vi "RobotMain.vi"() -> ()   [LabVIEW 2014]
uses:
  Command.ctl
  DataHighway.ctl
  <vilib>/userdefined/High Color/IMAQdx.ctl
  <vilib>/myRIO/Common/Instrument Driver Framework/myRIO v1.0/UART/vis/myRIO v1.0 Close UART.vi
  <vilib>/myRIO/Common/Instrument Driver Framework/Utilities/vis/FPGA Ref Manager.vi
  <vilib>/myRIO/Common/Instrument Driver Framework/myRIO v1.0/myRIO v1.0 Reset FPGA.vi
  <vilib>/myRIO/Common/Instrument Driver Framework/myRIO v1.0/IRQ/vis/myRIO v1.0 IRQ Info FGV.vi
  <vilib>/myRIO/Common/Instrument Driver Framework/myRIO v1.0/IRQ/vis/myRIO v1.0 Timer IRQ Info FGV.vi
  <vilib>/myRIO/Common/Instrument Driver Framework/myRIO v1.0/IRQ/vis/myRIO v1.0 ISR Agent.vi
  <vilib>/ErrorRing/Error Ring.xnode
  <vilib>/myRIO/Instrument Drivers/Utilities/Utilities.lvlib
  <vilib>/vision/driver/NI_Vision_Acquisition_Software.lvlib
panel:
  out "Camera open ok?":errorcluster
  out "Robot Run ok":bool
  out "Color Image":T1(plugin-control)
  out "BW Image":T1(plugin-control)
  out "Nb Circles":i32
  out "Camera Data":T2(array[cluster])
  out "GPS":cluster{"X pos":i32, "Y pos":i32, "Heading":dbl}
  in  "Tug Letter":string="T"
  out "GPS OK?":bool
  out "DataHWay":T3
  out "ComHWayFromOCU":T4 {"Speed" scale=-2.0..10.0; "Rudder" scale=-10.0..10.0}
  in  "stop robot control":bool
  out "Final myRIO error":errorcluster
  # "set\nletter"
  # "Robot will run headless\nwithout a control panel\nso keep this control panel\nas simple as possible while\nstill allowing debugging."
  # "Data Highway carries all robot data"
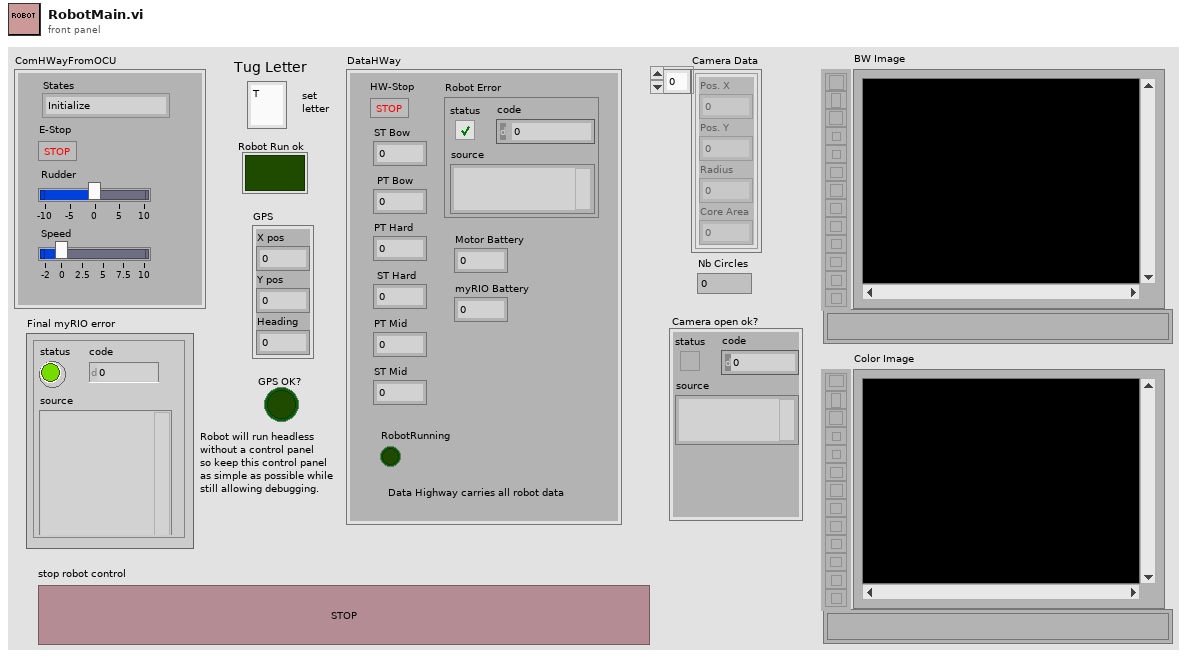
[diagram p1: front panel]
types:
  T1 = typedef "IMAQ Image.ctl" = refnum<image>
  T2 = cluster{"Pos. X":i32, "Pos. Y":i32, "Radius":i32, "Core Area":i32}[]
  T3 = typedef "DataHighway.ctl" = cluster{"HW-Stop":bool, "ST Bow":dbl, " PT Bow":dbl, "PT Hard":dbl, "RobotRunning":bool, "Robot Error":errorcluster, " ST Hard":dbl, "PT Mid":dbl, "ST Mid":dbl, "Motor Battery":dbl, "myRIO Battery":dbl}
  T4 = typedef "Command.ctl" = cluster{"States":enum16{"Initialize", "Wait for Event", "Debug Robot", "Run Robot", "Exit", "Plan"}, "E-Stop":bool, "Rudder":dbl, "Speed":dbl}
  T5 = typedef "IMAQdx.ctl" = refnum<k21>
  T6 = typedef "Image Type" = u32
  T7 = enum16{"Initialize", "Wait for Event", "Debug Robot", "Run Robot", "Exit"}
  T8 = enum16{"Initialize", "Wait for Event", "Debug Robot", "Run Robot", "Exit", "Plan"}
  T9 = cluster{"StarBow":dbl, "Portbow":dbl, "PortHard":dbl, "Starhard":dbl, "PortMid":dbl, "StarMid":dbl}
  T10 = cluster{"regular expression":string, i32, i32, i32}
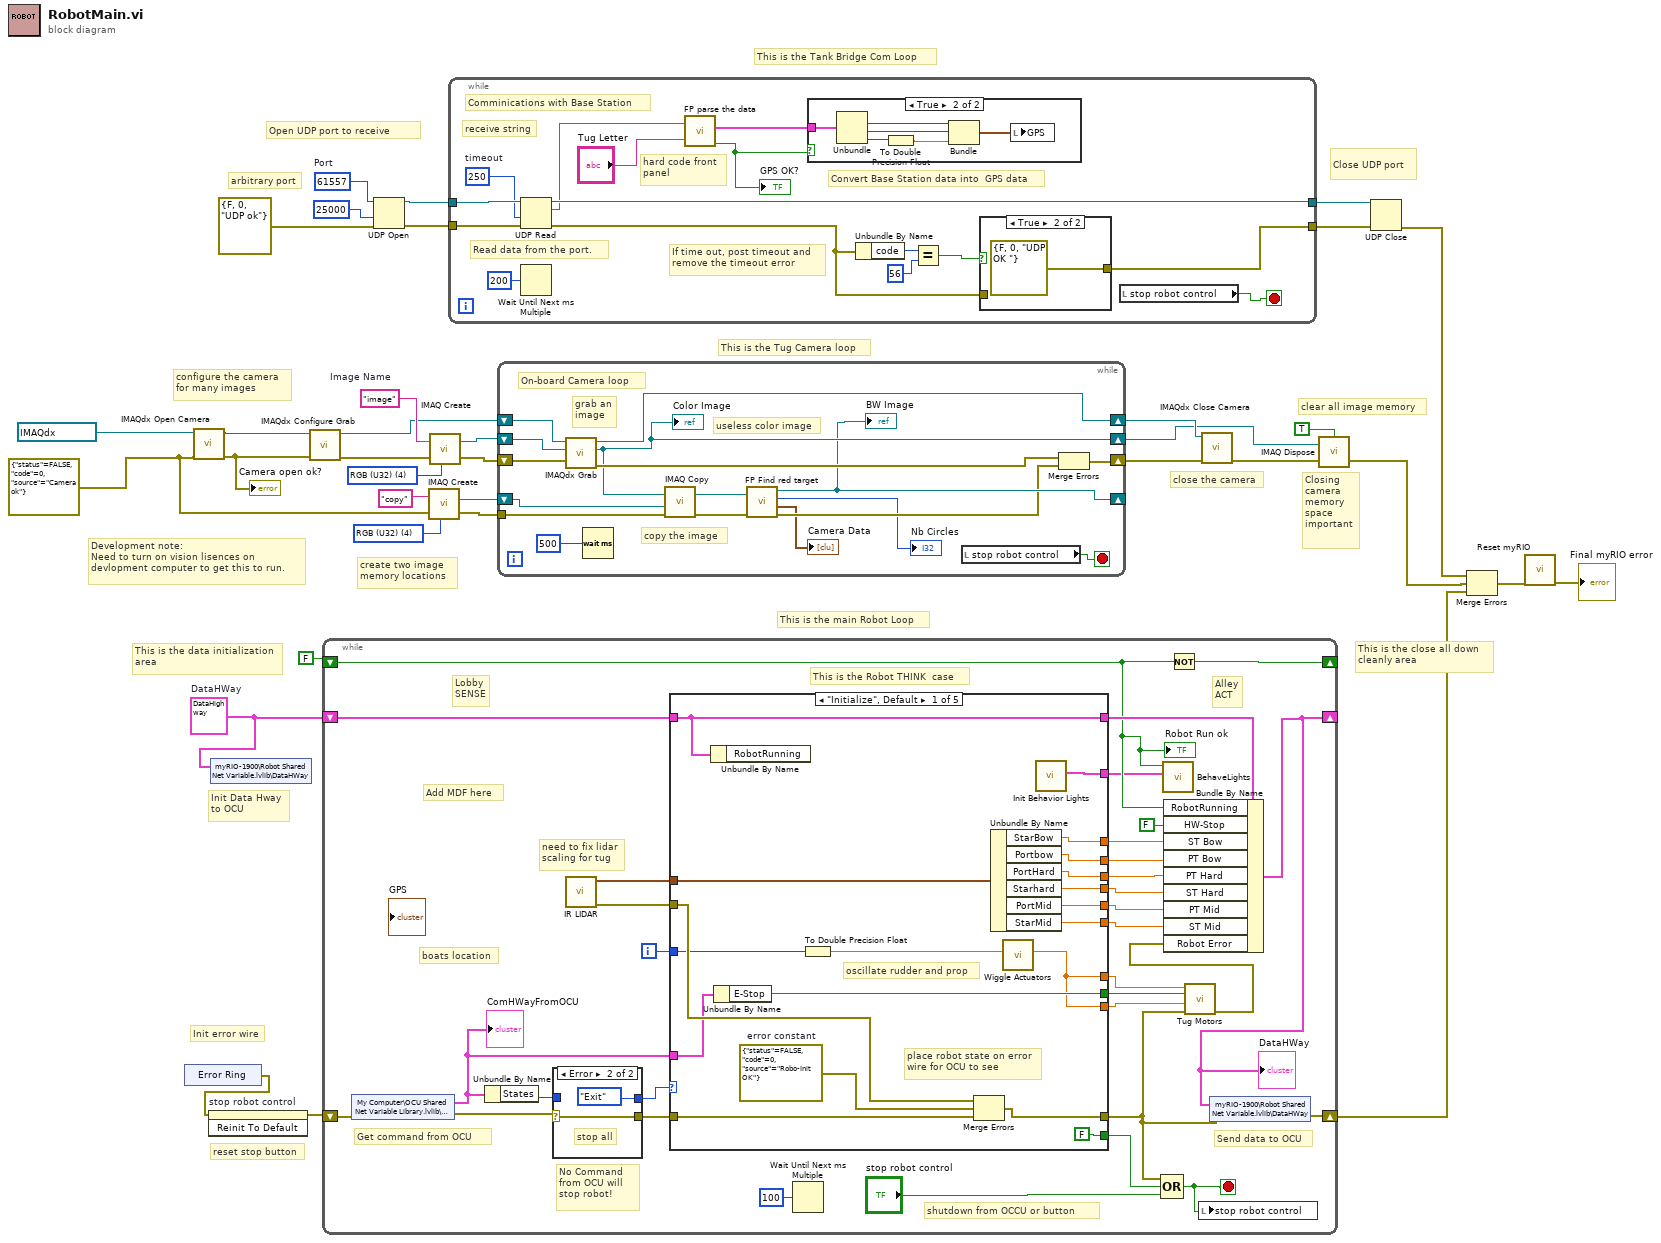
[diagram p0: block diagram]
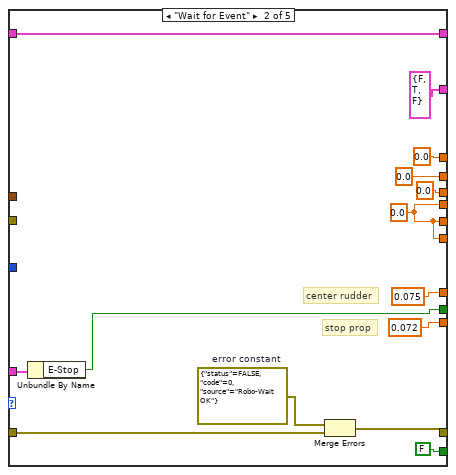
[diagram p5: hidden frame]
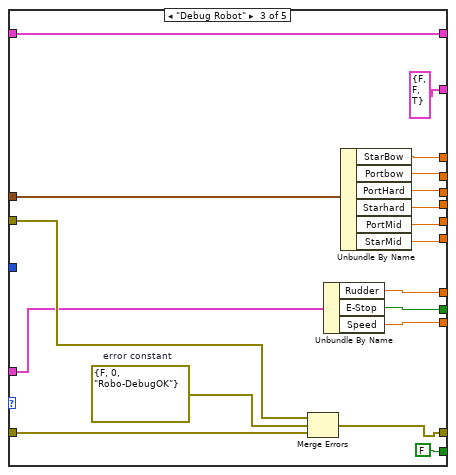
[diagram p6: hidden frame]
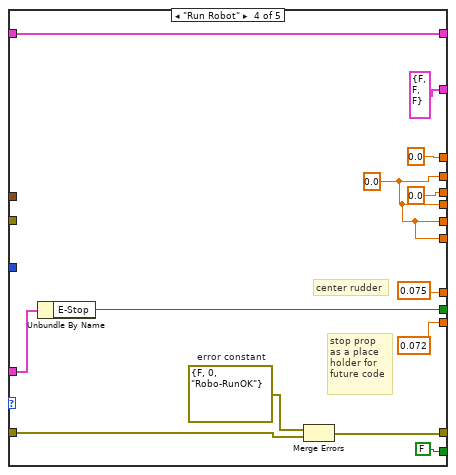
[diagram p7: hidden frame]
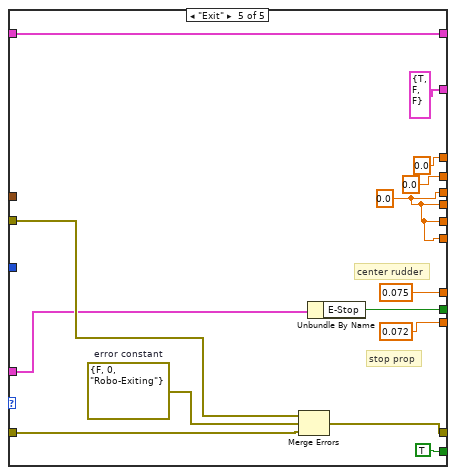
[diagram p8: hidden frame]
diagram:
  w23 = T6 4 items=["Grayscale (U8)", "Grayscale (I16)", "Grayscale (SGL)", "Complex (CSG)", "RGB (U32)", "HSL (U32)", "RGB (U64)", "Grayscale (U16)"] ("Image Type")
  w1 = errorcluster {"status"=FALSE, "code"=0, "source"="Camera ok"} ("error in")
  w21 = T6 4 items=["Grayscale (U8)", "Grayscale (I16)", "Grayscale (SGL)", "Complex (CSG)", "RGB (U32)", "HSL (U32)", "RGB (U64)", "Grayscale (U16)"] ("Image Type")
  w22 = "image"  # Image Name
  w29 = u16 61557  # Port
  w34 = T3 {"HW-Stop"=FALSE, "ST Bow"=0.0, " PT Bow"=0.0, "PT Hard"=0.0, "RobotRunning"=FALSE, "Robot Error"={"status"=FALSE, "code"=0, "source"=""}, " ST Hard"=0.0, "PT Mid"=0.0, "ST Mid"=0.0, "Motor Battery"=0.0, "myRIO Battery"=0.0}  # DataHWay
  # "Development note:\nNeed to turn on vision lisences on \ndevlopment computer to get this to run."
  # "create two image\nmemory locations"
  # "Closing \ncamera\nmemory\nspace\nimportant"
  # "This is the Tug Camera loop"
  # "clear all image memory"
  # "close the camera"
  # "configure the camera\nfor many images"
  # "arbitrary port"
  # "This is the Tank Bridge Com Loop"
  # "Close UDP port"
  # "Open UDP port to receive"
  # "reset stop button"
  # "Init error wire"
  # "Init Data Hway\nto OCU"
  # "This is the close all down \ncleanly area"
  # "This is the data initialization\narea"
  # "This is the main Robot Loop"
  n1 = xnode "Error Ring"() -> ("error out"=w33:errorcluster)
  n2 = call <vilib>:"IMAQdx Open Camera.vi"("error in"=w1, "Session In"=T5 "cam0") -> ("error out"=w6:errorcluster, "Session Out"=w7:T5)  [unwired: 8 in]
  "Camera open ok?" <- w6
  n3 = invoke on="stop robot control" class="Bool (strict)" method="Reinit To Default"(error in=w33) -> (error out=w32:errorcluster)  [unwired: 2 in, 2 out]
  n4 = shared-variable "myRIO-1900\\Robot Shared Net Variable.lvlib\\DataHWay"(w34) -> ()  [unwired: 1 in, 1 out]
  n5 = call <vilib>:"IMAQdx Configure Grab.vi"("error in"=w6, "Session In"=w7) -> ("error out"=w20:errorcluster, "Session Out"=w17:T5)  [unwired: 8 out]
  n6 = while {
    shift-right: [w59] -> w4
    shift-left: w32 -> [w56]
    shift-right: [w54] -> _
    shift-left: w34 -> [w63]
    shift-right: [w58] -> _
    shift-left: FALSE -> [w52]
    i -> [w41]
    stop <- w36 stop-if-true
    # "boats location"
    # "Add MDF here"
    # "need to fix lidar\nscaling for tug"
    # "No Command \nfrom OCU will\nstop robot!"
    # "Get command from OCU"
    # "Send data to OCU"
    # "shutdown from OCCU or button"
    # "Alley\nACT"
    # "This is the Robot THINK  case"
    # "Lobby\nSENSE"
    n7 = shared-variable "My Computer\\OCU Shared Net Variable Library.lvlib\\ComHWay"(error in=w56) -> (w60:T4, error out=w55:errorcluster)
    "ComHWayFromOCU" <- w60
    n8 = Unbundle By Name(w60) -> ("States"=w61:T8)
    n9 = case shown="Error" w55 {
      selector: w55 -> [w69 w71]
      tunnel: [w69 w71] -> w66
      tunnel: [w68 T7."Exit" ("States")] -> w67
      tunnel: w61 -> [w68 _]
      frame No Error {
      }
      frame Error {
        # "stop all"
      }
    }
    n10 = call "IR LIDAR.vi"() -> ("error out"=w49:errorcluster, "Range"=w50:T9)  [unwired: 10 in]
    n11 = case shown="\"Initialize\", Default" w67 {
      tunnel: w66 -> [w89 w102 w120 w133 w147]
      tunnel: [w88 w101 w119 w132 w146] -> w45
      tunnel: [FALSE FALSE FALSE FALSE TRUE] -> w65
      tunnel: w63 -> [w86 w103 w122 w135 w148]
      tunnel: [w86 w103 w122 w135 w148] -> w57
      tunnel: w60 -> [w79 w95 w111 w127 w140]
      tunnel: [w85 cluster{"Red":bool, "Blue":bool, "Green":bool} {"Red"=FALSE, "Blue"=TRUE, "Green"=FALSE} ("Lights Out") cluster{"Red":bool, "Blue":bool, "Green":bool} {"Red"=FALSE, "Blue"=FALSE, "Green"=TRUE} ("Lights Out") cluster{"Red":bool, "Blue":bool, "Green":bool} {"Red"=FALSE, "Blue"=FALSE, "Green"=FALSE} ("Lights Out") cluster{"Red":bool, "Blue":bool, "Green":bool} {"Red"=TRUE, "Blue"=FALSE, "Green"=FALSE} ("Lights Out")] -> w51
      tunnel: w50 -> [w83 _ w116 _ _]
      tunnel: w49 -> [w84 _ w112 _ w141]
      tunnel: [w82 0.0 ("Port") w115 0.0 ("Port") 0.0 ("Port")] -> w48
      tunnel: [w81 0.0 ("Center") w114 w123 0.0 ("Center")] -> w47
      tunnel: [w80 0.0 ("Starboard") w113 0.0 ("Starboard") w136] -> w46
      tunnel: [w75 0.075 ("Rudder") w110 0.075 ("Rudder") 0.075 ("Rudder")] -> w44
      tunnel: [w78 w94 w109 w126 w139] -> w43
      tunnel: [w75 0.072 ("Speed") w108 0.072 ("Speed") 0.072 ("Speed")] -> w42
      tunnel: w41 -> [w77 _ _ _ _]
      tunnel: [w74 w91 w107 w123 w136] -> w39
      tunnel: [w73 w91 w106 w123 w136] -> w38
      tunnel: [w72 w91 w105 w123 w136] -> w37
      frame "Initialize", Default {
        w87 = errorcluster {"status"=FALSE, "code"=0, "source"="Robo-Init OK"}  # error constant
        # "oscillate rudder and prop"
        # "place robot state on error\nwire for OCU to see"
        n12 = Unbundle By Name "Unbundle By Name"(w86) -> ()  [unwired: 1 out]
        n13 = Unbundle By Name(w79) -> ("E-Stop"=w78:bool)
        n14 = To Double Precision Float(number=w77) -> (double precision float=w76:dbl)
        n15 = Merge Errors "Merge Errors"(w84, w87, w89) -> (w88:errorcluster)
        n16 = Unbundle By Name(w83) -> ("StarBow"=w82:dbl, "Portbow"=w81:dbl, "PortHard"=w80:dbl, "Starhard"=w74:dbl, "PortMid"=w73:dbl, "StarMid"=w72:dbl)
        n17 = call "Wiggle Actuators.vi"("Trigger"=w76) -> ("MotorCommand"=w75:dbl)  [unwired: 10 in]
        n18 = call "Init Behavior Lights.vi"() -> ("Lights Out"=w85:cluster{"Red":bool, "Blue":bool, "Green":bool})  [unwired: 11 in]
      }
      frame "Wait for Event" {
        w91 = 0.0 ("Starhard")
        w100 = errorcluster {"status"=FALSE, "code"=0, "source"="Robo-Wait OK"}  # error constant
        # "stop prop"
        # "center rudder"
        n19 = Unbundle By Name(w95) -> ("E-Stop"=w94:bool)
        n20 = Merge Errors "Merge Errors"(w100, w102) -> (w101:errorcluster)
      }
      frame "Debug Robot" {
        w118 = errorcluster {"status"=FALSE, "code"=0, "source"="Robo-DebugOK"}  # error constant
        n21 = Merge Errors "Merge Errors"(w112, w118, w120) -> (w119:errorcluster)
        n22 = Unbundle By Name "Unbundle By Name"(w111) -> ("Rudder"=w110:dbl, "E-Stop"=w109:bool, "Speed"=w108:dbl)
        n23 = Unbundle By Name(w116) -> ("StarBow"=w115:dbl, "Portbow"=w114:dbl, "PortHard"=w113:dbl, "Starhard"=w107:dbl, "PortMid"=w106:dbl, "StarMid"=w105:dbl)
      }
      frame "Run Robot" {
        w123 = 0.0 ("Center")
        w131 = errorcluster {"status"=FALSE, "code"=0, "source"="Robo-RunOK"}  # error constant
        # "stop prop\nas a place\nholder for\nfuture code"
        # "center rudder"
        n24 = Unbundle By Name(w127) -> ("E-Stop"=w126:bool)
        n25 = Merge Errors "Merge Errors"(w131, w133) -> (w132:errorcluster)
      }
      frame "Exit" {
        w136 = 0.0 ("Starboard")
        w145 = errorcluster {"status"=FALSE, "code"=0, "source"="Robo-Exiting"}  # error constant
        # "stop prop"
        # "center rudder"
        n26 = Merge Errors "Merge Errors"(w141, w145, w147) -> (w146:errorcluster)
        n27 = Unbundle By Name(w140) -> ("E-Stop"=w139:bool)
      }
    }
    n28 = Wait Until Next ms Multiple(millisecond multiple=u32 100) -> ()  [unwired: 1 out]
    n29 = Compound Arithmetic op=OR(w45, w65, "stop robot control") -> (w36:bool)
    n30 = call "BehaveLights.vi"("BehLightIn"=w51, "Blink"=w52) -> ()  [unwired: 9 in, 1 out]
    n31 = Not(x=w52) -> (.not. x?=w58:bool)
    n32 = call "Tug Motors.vi"("error in (no error)"=w45, "Prop Speed"=w42, "MotorStop"=w43, "Rud Angle"=w44) -> ("error out"=w40:errorcluster)  [unwired: 7 in]
    n33 = Bundle By Name(cluster=w57, "RobotRunning"=w52, "HW-Stop"=FALSE, "ST Bow"=w48, "PT Bow"=w47, "PT Hard"=w46, "ST Hard"=w39, "PT Mid"=w38, "ST Mid"=w37, "Robot Error"=w40) -> (w54:T3)
    "DataHWay" <- w54
    n34 = local write "stop robot control"(w36) -> ()
    n35 = shared-variable "myRIO-1900\\Robot Shared Net Variable.lvlib\\DataHWay"(w54, error in=w45) -> (error out=w59:errorcluster)
    "Robot Run ok" <- w52
  }
  n36 = UDP Open(8:errorcluster {"status"=FALSE, "code"=0, "source"="UDP ok"} ("error in"), 9:25000 ("timeout ms (25000)"), 11:w29) -> (port=w28:refnum<k16>, 0:w27:errorcluster)  [unwired: 2 in, 1 out]
  n37 = call "IMAQ Create"("Image Name"="copy", "Image Type"=w23, "error in (no error)"=w1) -> ("New Image"=w14:T1, "error out"=w13:errorcluster)  [unwired: 2 in]
  n38 = call "IMAQ Create"("Image Name"=w22, "Image Type"=w21, "error in (no error)"=w20) -> ("New Image"=w16:T1, "error out"=w15:errorcluster)  [unwired: 1 in, 1 out]
  n39 = while {
    tunnel: w27 -> [w164]
    tunnel: w28 -> [w163]
    tunnel: [w162] -> w26
    tunnel: [w157] -> w25
    stop <- w150 stop-if-true
    w156 = 250  # timeout
    # "hard code front\npanel"
    # "Convert Base Station data into  GPS data"
    # "Comminications with Base Station"
    # "receive string"
    # "If time out, post timeout and\nremove the timeout error"
    # "Read data from the port."
    n40 = UDP Read(connection ID=w163, timeout ms (25000)=w156, 8:w164) -> (data out=w152:string, error out=w158:errorcluster, 3:w162:refnum<k16>)  [unwired: 1 in, 2 out]
    n41 = Wait Until Next ms Multiple(millisecond multiple=u32 200) -> ()  [unwired: 1 out]
    n42 = call "FP parse the data.vi"("Nav String"=w152, "Tug"="Tug Letter") -> ("Tug Location"=w153:T10, "Valid?"=w151:bool)  [unwired: 2 out]
    "GPS OK?" <- w151
    n43 = case shown="True" w151 {
      tunnel: w153 -> [_ w170]
      frame False {
      }
      frame True {
        n44 = Unbundle(w170) -> (w169:i32, w168:i32, w166:i32)  [unwired: 1 out]
        n45 = To Double Precision Float(number=w166) -> (double precision float=w167:dbl)
        n46 = Bundle(w169, w168, w167) -> (w165:cluster{i32, i32, dbl})  [unwired: 1 in]
        n47 = local write "GPS"(w165) -> ()
      }
    }
    n48 = Unbundle By Name(w158) -> ("code"=w161:i32)
    n49 = Equal?(x=w161, y=56) -> (x = y?=w159:bool)
    n50 = case shown="True" w159 {
      tunnel: [w171 errorcluster {"status"=FALSE, "code"=0, "source"="UDP OK "} ("error out")] -> w157
      tunnel: w158 -> [w171 _]
      frame False {
      }
      frame True {
      }
    }
    n51 = local read "stop robot control"() -> (w150:bool)
  }
  n52 = while {
    shift-right: [w182] -> w10
    shift-left: w15 -> [w180]
    shift-right: [w181] -> w11
    shift-left: w16 -> [w189]
    shift-right: [w184] -> w12
    shift-left: w17 -> [w188]
    tunnel: w13 -> [w186]
    shift-right: [w177] -> _
    shift-left: w14 -> [w185]
    stop <- w174 stop-if-true
    # "useless color image"
    # "grab an\nimage"
    # "copy the image"
    # "On-board Camera loop"
    n53 = call <vilib>:"IMAQdx Grab.vi"("error in"=w180, "Image In"=w189, "Session In"=w188) -> ("error out"=w183:errorcluster, "Image Out"=w181:T1, "Session Out"=w184:T5)  [unwired: 5 in, 1 out]
    "Color Image" <- w181
    n54 = Wait (ms)(milliseconds to wait=u32 500) -> ()  [unwired: 1 out]
    n55 = call "IMAQ Copy"("error in (no error)"=w186, "Image Dst"=w185, "Image Src"=w181) -> ("error out"=w178:errorcluster, "Image Dst Out"=w179:T1)  [unwired: 3 in]
    n56 = call "FP Find red target.vi"("Image In"=w179, "error in (no error)"=w178) -> ("Image Dst Out"=w177:T1, "Nb Circles (Circle Detection 1)"=→"Nb Circles":i32, "Camera Data"=→"Camera Data":T2, "error out"=w176:errorcluster)
    "BW Image" <- w177
    n57 = local read "stop robot control"() -> (w174:bool)
    n58 = Merge Errors(w183, w176) -> (w182:errorcluster)
  }
  n59 = call <vilib>:"IMAQdx Close Camera.vi"("error in"=w10, "Session In"=w12) -> ("error out"=w18:errorcluster)  [unwired: 9 out]
  n60 = call "IMAQ Dispose"("All Images? (No)"=TRUE, "Image"=w11, "error in (no error)"=w18) -> ("error out"=w8:errorcluster)  [unwired: 3 out]
  n61 = UDP Close(connection ID=w26, 8:w25) -> (error out=w9:errorcluster)  [unwired: 1 out]
  n62 = Merge Errors(w9, w8, w4) -> (w3:errorcluster)
  n63 = call <vilib>:"Reset myRIO.vi"("error in (no error)"=w3) -> ("error out"=→"Final myRIO error":errorcluster)  [unwired: 10 in]
